vi "sc5511a_get_device_info.vi"(0 "deviceHandle":u32 format="%.0x", 5 "error in":errorcluster) -> (14 "deviceHandle":u32 format="%.0x", 16 "Device Info":T1 {"Product SN" format="%.0x"; "Hardware Rev" format="%.2g"; "Firmware Rev" format="%.2g"}, 19 "error out":errorcluster)   [LabVIEW 2010]
uses:
  sc5511a_rs232.dll
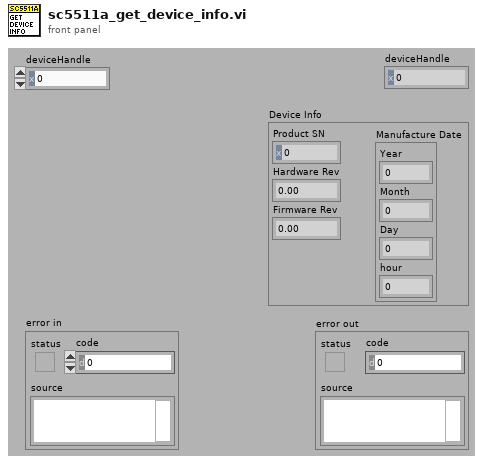
[diagram p1: front panel]
types:
  T1 = cluster{"Product SN":u32, "Hardware Rev":sgl, "Firmware Rev":sgl, "Manufacture Date":cluster{"Year":u8, "Month":u8, "Day":u8, "hour":u8}}
  T2 = cluster{"Year":u8, "Month":u8, "Day":u8, "hour":u8}
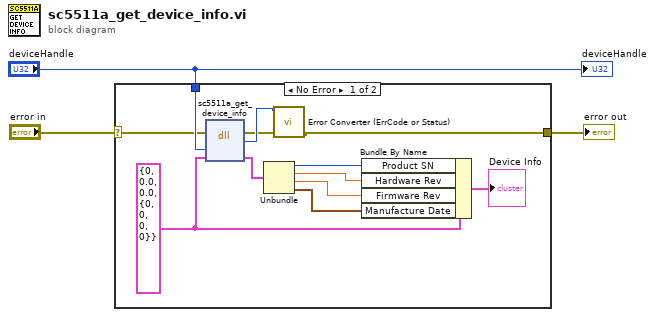
[diagram p0: block diagram]
diagram:
  n1 = case shown="No Error" "error in" {
    selector: "error in" -> [w4 w16]
    tunnel: [w14 w16] -> w2
    tunnel: "deviceHandle" -> [w11 _]
    frame No Error {
      w7 = T1 {"Product SN"=0, "Hardware Rev"=0.0, "Firmware Rev"=0.0, "Manufacture Date"={"Year"=0, "Month"=0, "Day"=0, "hour"=0}} ("Device Info")
      n2 = dll-call lib="sc5511a_rs232.dll" fn="sc5511a_get_device_info"(error in=w4, "deviceHandle"=w11, "device_info"=w7) -> (error out=w13:errorcluster, "return type"=w15:i32, "device_info"=w12:T1)  [unwired: 3 in, 1 out]
      n3 = Unbundle(w12) -> ("Product SN"=w10:u32, "Hardware Rev"=w9:sgl, "Firmware Rev"=w8:sgl, "Manufacture Date"=w6:T2)
      n4 = call "Error Converter (ErrCode or Status).vi"("error in (no error)"=w13, "error code"=w15) -> ("error out"=w14:errorcluster)  [unwired: 9 in]
      n5 = Bundle By Name(cluster=w7, "Product SN"=w10, "Hardware Rev"=w9, "Firmware Rev"=w8, "Manufacture Date"=w6) -> (→"Device Info":T1)
    }
    frame Error {
    }
  }
  "error out" <- w2
  "deviceHandle" <- "deviceHandle"
